vi "Dispach PVMonitors.vi"(8 "Error In":errorcluster, 11 "CS++ControllerActor in":refnum<class "CS++ControllerActor.lvclass">) -> (0 "Error Out":errorcluster, 3 "CS++ControllerActor out":refnum<class "CS++ControllerActor.lvclass">)   [LabVIEW 2014, in "CS++ControllerActor.lvlib" / "CS++ControllerActor.lvclass"]
doc: "Dispatch nested PVMonitor actors according to PV protocoll prefix."
uses:
  CS++ControllerActor.lvclass
  CS++PVMonitor/CS++PVMonitor.lvclass
  CS++GUIActor Messages/Update-PV Msg/Update-PV Msg.lvclass
  CS++BaseActor/CS++BaseActor.lvclass/CS++BaseActor.ctl
  CS++PVMonitor Messages/CS++PVUpdate Msg/CS++PVUpdate Msg.lvclass/CS++PVUpdate Msg.ctl
  Classes/CS++ProcessVariables/ProcessVariable/PV.lvclass/PV.ctl
  Libraries/Base/FGV Action.ctl
  CS++PVMonitor Messages/Register PVs Msg/Register PVs Msg.lvclass/Register PVs Msg.ctl
  <vilib>/ActorFramework/Message Enqueuer/Message Enqueuer.lvclass/Message Enqueuer.ctl
  CS++ControllerActor.lvclass/CS++ControllerActor.ctl
  CS++BaseActor/Read Object Name.vi
  <vilib>/ActorFramework/Message Enqueuer/Enqueue.vi
  <vilib>/ActorFramework/Message Priority Queue/Priority Enqueue.vi
  CS++PVMonitor Messages/CS++PVUpdate Msg/CS++PVUpdate Msg.lvclass
  Classes/CS++ProcessVariables/PVConnection/PVConnection.lvclass
  Classes/CS++ProcessVariables/ProcessVariable/PV.lvclass
  <vilib>/ActorFramework/Message Enqueuer/Message Enqueuer.lvclass
  CS++PVMonitor Messages/Register PVs Msg/Register PVs Msg.lvclass
  CS++BaseActor/CS++BaseActor.lvclass
  <vilib>/ActorFramework/Actor/Actor.lvclass
  Libraries/Base/CS++Base.lvlib
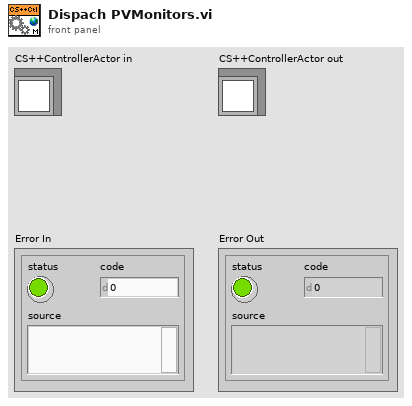
[diagram p1: front panel]
types:
  T1 = cluster{"Msgs":refnum<class "Update-PV Msg.lvclass">[]}[]
  T2 = typedef "CS++Base.lvlib/FGV Action.ctl" = enum16{"add", "replace", "read", "remove", "reset", "get attributes"}
  T3 = cluster{"Name":string, "Polling-String":string, "CS++PVUpdate Msg":refnum<class "CS++PVUpdate Msg.lvclass">, "PVConnection":refnum<class "PVConnection.lvclass">}[]
  T4 = cluster{"Msgs":refnum<class "CS++PVUpdate Msg.lvclass">[]}
  T5 = cluster{"Msgs":refnum<class "CS++PVUpdate Msg.lvclass">[]}[]
  T6 = cluster{refnum<class "CS++PVUpdate Msg.lvclass">[]}
  T7 = cluster{"Accessors:Device Actor's Enqueuer":refnum<class "Message Enqueuer.lvclass">, "Msgs":refnum<class "CS++PVUpdate Msg.lvclass">[]}
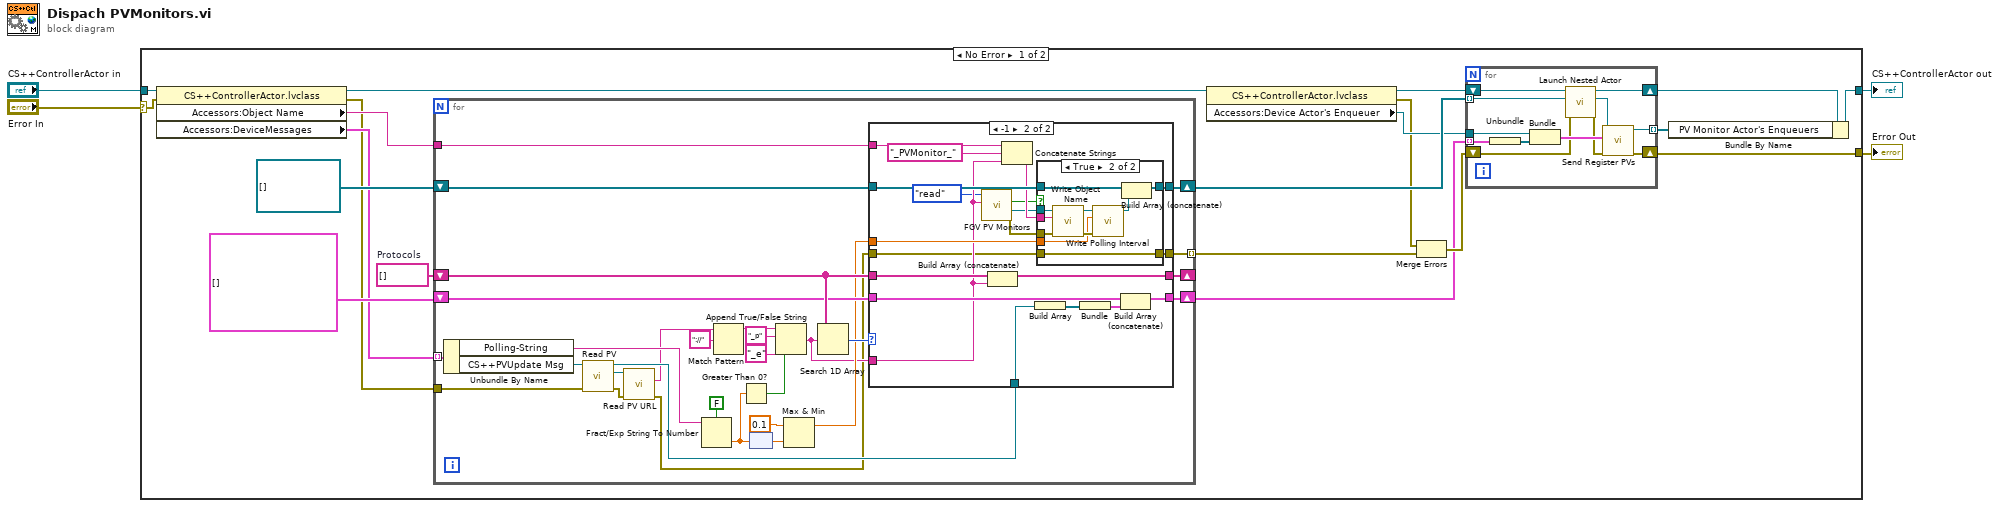
[diagram p0: block diagram]
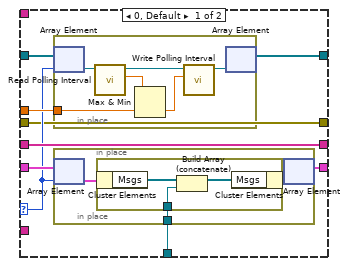
[diagram p2: hidden frame]
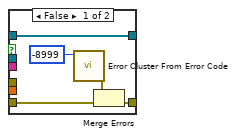
[diagram p3: hidden frame]
diagram:
  n1 = case shown="No Error" "Error In" {
    selector: "Error In" -> [w20 w123]
    tunnel: [w21 w123] -> w3
    tunnel: [w22 w122] -> w1
    tunnel: "CS++ControllerActor in" -> [w23 w122]
    frame No Error {
      w17 = string[] []  # Protocols
      n2 = property class="CS++ControllerActor.lvclass"(reference=w23, error in=w20) -> (reference out=w7:refnum<class "CS++ControllerActor.lvclass">, error out=w5:errorcluster, "Accessors:Object Name"=w11:string, "Accessors:DeviceMessages"=w6:T3)
      n3 = for {
        shift-right: [w65] -> w16
        shift-left: refnum<class "CS++PVMonitor.lvclass">[] [] -> [w62]
        shift-right: [w64] -> _
        shift-left: w17 -> [w63]
        tunnel: w11 -> [w61]
        shift-right: [w59] -> w13
        shift-left: T1 [] -> [w60]
        tunnel: [w58] -> w12 mode=indexing
        tunnel: w6 -> [w45] mode=indexing
        tunnel: w5 -> [w37]
        n4 = Unbundle By Name(w45) -> ("Polling-String"=w44:string, "CS++PVUpdate Msg"=w43:refnum<class "CS++PVUpdate Msg.lvclass">)
        n5 = call "Read PV.vi"("error in (no error)"=w37, "CS++PVUpdate Msg in"=w43) -> ("error out"=w39:errorcluster, "PV"=w41:refnum<class "PV.lvclass">, "CS++PVUpdate Msg out"=w42:refnum<class "CS++PVUpdate Msg.lvclass">)  [unwired: 7 in]
        n6 = call "Read PV URL.vi"("error in (no error)"=w39, "PV in"=w41) -> ("error out"=w38:errorcluster, "PV URL"=w40:string)  [unwired: 7 in, 1 out]
        n7 = Fract/Exp String To Number(use system decimal point (T)=FALSE, string=w44) -> (number=w52:dbl)  [unwired: 2 in, 1 out]
        n8 = Match Pattern(string=w40, regular expression="://") -> (before substring=w50:string)  [unwired: 1 in, 3 out]
        n9 = Greater Than 0?(x=w52) -> (x > 0?=w48:bool)
        n10 = node(w52) -> (w54:dbl[unit])
        n11 = Append True/False String(1:w48, 2:"_e" ("false string"), 3:"_p" ("true string"), 4:w50) -> (0:w49:string)
        n12 = Max & Min(x=dbl[unit] 0.1, y=w54) -> (max(x,y)=w51:dbl[unit])  [unwired: 1 out]
        n13 = Search 1D Array(1D array=w63, element=w49) -> (index of element=w55:i32)  [unwired: 1 in]
        n14 = case shown="-1" w55 {
          selector: w55 -> [w69 _]
          tunnel: [w72 w106] -> w65
          tunnel: [w74 w105] -> w64
          tunnel: w49 -> [_ w93]
          tunnel: w63 -> [w74 w104]
          tunnel: w62 -> [w73 w103]
          tunnel: w51 -> [w71 w100]
          tunnel: w61 -> [_ w99]
          tunnel: w42 -> [w68 w98]
          tunnel: w60 -> [w70 w96]
          tunnel: [w67 w94] -> w59
          tunnel: w38 -> [w66 w89]
          tunnel: [w66 w87] -> w58
          frame 0, Default {
            n15 = in-place {
              in-place-border: w71 -> [w84]
              n16 = in-place-array #1(w73, w69) -> (w86:refnum<class "CS++PVMonitor.lvclass">)
              n17 = call "Read Polling Interval.vi"("CS++BaseActor in"=w86) -> ("Polling Interval"=w85:dbl[unit], "CS++BaseActor out"=w83:refnum<class "CS++PVMonitor.lvclass">)  [unwired: 8 in, 1 out]
              n18 = Max & Min(x=w85, y=w84) -> (min(x,y)=w82:dbl[unit])  [unwired: 1 out]
              n19 = call "Write Polling Interval.vi"("Polling Interval"=w82, "CS++BaseActor in"=w83) -> ("CS++BaseActor out"=w81:refnum<class "CS++PVMonitor.lvclass">)  [unwired: 8 in, 1 out]
              n20 = in-place-array #1(w81) -> (w72:refnum<class "CS++PVMonitor.lvclass">[])  [unwired: 1 out]
            }
            n21 = in-place {
              in-place-border: w68 -> [w75]
              n22 = in-place-array #2(w70, w69) -> (w77:T4)
              n23 = in-place {
                in-place-border: w75 -> [w79]
                n24 = in-place-cluster #3(w77) -> ("Msgs"=w80:refnum<class "CS++PVUpdate Msg.lvclass">[])
                n25 = Build Array (concatenate)(w80, w79) -> (w78:refnum<class "CS++PVUpdate Msg.lvclass">[])
                n26 = in-place-cluster #3("Msgs"=w78) -> (w76:T4)
              }
              n27 = in-place-array #2(w76) -> (w67:T5)  [unwired: 1 out]
            }
          }
          frame -1 {
            n28 = call "FGV PV Monitors.vi"("PV Monitor"=w93, "Action (read)"=FGV_Action."read") -> ("Error Out"=w90:errorcluster, "CS++PVMonitor"=w92:refnum<class "CS++PVMonitor.lvclass">, "Success"=w88:bool)  [unwired: 5 in, 2 out]
            n29 = Build Array (concatenate)(w104, w93) -> (w105:string[])
            n30 = Concatenate Strings(w99, "_PVMonitor_" ("Object Name"), w93) -> (w101:string)
            n31 = Build Array(w98) -> (w97:refnum<class "CS++PVUpdate Msg.lvclass">[])
            n32 = case shown="True" w88 {
              tunnel: [w111 w121] -> w106
              tunnel: w103 -> [w111 w120]
              tunnel: w101 -> [_ w119]
              tunnel: w100 -> [_ w116]
              tunnel: w92 -> [_ w114]
              tunnel: w90 -> [_ w113]
              tunnel: w89 -> [w110 w112]
              tunnel: [w109 w112] -> w87
              frame False {
                n33 = call <vilib>:"Error Cluster From Error Code.vi"("error code (0)"=-8999) -> ("error out"=w108:errorcluster)  [unwired: 8 in]
                n34 = Merge Errors(w108, w110) -> (w109:errorcluster)
              }
              frame True {
                n35 = call "Write Object Name.vi"("error in (no error)"=w113, "Object Name"=w119, "CS++BaseActor in"=w114) -> ("error out"=w117:errorcluster, "CS++BaseActor out"=w118:refnum<class "CS++PVMonitor.lvclass">)  [unwired: 7 in]
                n36 = call "Write Polling Interval.vi"("error in (no error)"=w117, "Polling Interval"=w116, "CS++BaseActor in"=w118) -> ("CS++BaseActor out"=w115:refnum<class "CS++PVMonitor.lvclass">)  [unwired: 7 in, 1 out]
                n37 = Build Array (concatenate)(w120, w115) -> (w121:refnum<class "CS++PVMonitor.lvclass">[])
              }
            }
            n38 = Bundle(w97) -> (w95:T6)  [unwired: 1 in]
            n39 = Build Array (concatenate)(w96, w95) -> (w94:T5)
          }
        }
      }
      n40 = property class="CS++ControllerActor.lvclass"(reference=w7) -> (reference out=w10:refnum<class "CS++ControllerActor.lvclass">, error out=w8:errorcluster, "Accessors:Device Actor's Enqueuer"=w9:refnum<class "Message Enqueuer.lvclass">)  [unwired: 1 in]
      n41 = Merge Errors(w8, w12) -> (w15:errorcluster)
      n42 = for {
        tunnel: w9 -> [w35]
        tunnel: w16 -> [w26] mode=indexing
        tunnel: w13 -> [w30] mode=indexing
        tunnel: [w27] -> w19 mode=indexing
        shift-right: [w28] -> w21
        shift-left: w15 -> [w32]
        shift-right: [w31] -> w24
        shift-left: w10 -> [w29]
        n43 = Unbundle(w30) -> ("Msgs"=w25:refnum<class "CS++PVUpdate Msg.lvclass">[])
        n44 = Bundle("Accessors:Device Actor's Enqueuer"=w35, "Msgs"=w25) -> (w34:T7)  [unwired: 1 in]
        n45 = call <vilib>:"Launch Nested Actor.vi"("error in (no error)"=w32, "Nested Actor"=w26, "Caller Actor in"=w29) -> ("error out"=w33:errorcluster, "Nested Actor's Enqueuer"=w36:refnum<class "Message Enqueuer.lvclass">, "Caller Actor out"=w31:refnum<class "CS++ControllerActor.lvclass">)  [unwired: 6 in]
        n46 = call "Send Register PVs.vi"("error in (no error)"=w33, "Register Info"=w34, "Message Enqueuer"=w36) -> ("error out"=w28:errorcluster, "Message Enqueuer out"=w27:refnum<class "Message Enqueuer.lvclass">)  [unwired: 7 in]
      }
      n47 = Bundle By Name(cluster=w24, "PV Monitor Actor's Enqueuers"=w19) -> (w22:refnum<class "CS++ControllerActor.lvclass">)
    }
    frame Error {
    }
  }
  "Error Out" <- w3
  "CS++ControllerActor out" <- w1
